vi "Error Builder.vi"(8 "error in (no error)":errorcluster, 10 "This VI":refnum<vi>, 11 "Optris PI in":refnum<class "Optris PI.lvclass">) -> (0 "Error out":errorcluster, 3 "Optris PI out":refnum<class "Optris PI.lvclass">)   [LabVIEW 2018, in "Optris PI.lvlib" / "Optris PI.lvclass"]
uses:
  Optris PI.lvclass
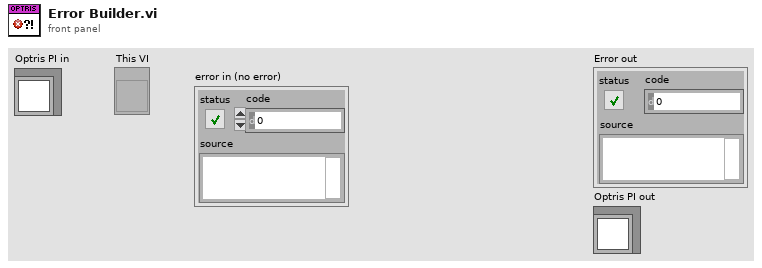
[diagram p1: front panel]
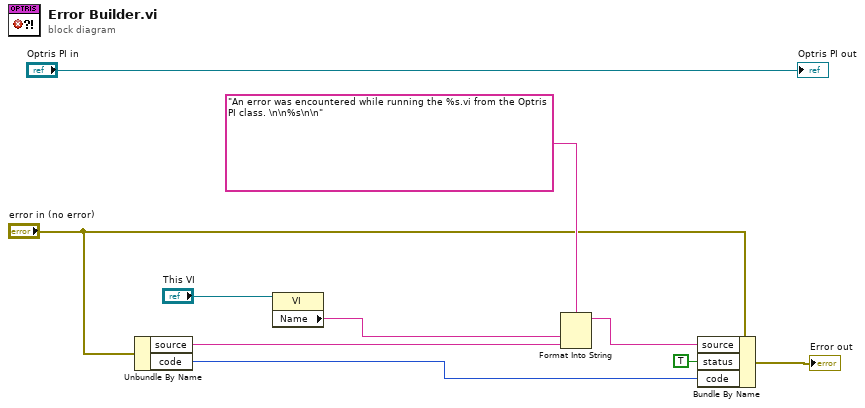
[diagram p0: block diagram]
diagram:
  n1 = Unbundle By Name("error in (no error)") -> ("source"=w6:string, "code"=w7:i32)
  n2 = property class="VI"(reference="This VI") -> ("Name"=w2:string)  [unwired: 1 in, 2 out]
  n3 = Format Into String(format string="An error was encountered while running the %s.vi from the Optris PI class. \n\n%s\n\n", w2, w6) -> (resulting string=w9:string)  [unwired: 2 in, 1 out]
  n4 = Bundle By Name(cluster="error in (no error)", "source"=w9, "status"=TRUE, "code"=w7) -> (→"Error out":errorcluster)
  "Optris PI out" <- "Optris PI in"
